vi "Day 3 - Rucksack Reorganization.vi"() -> ()   [LabVIEW 2020, in "AoC 2022.lvlib"]
uses:
  AoC 2022.lvlib
  ce42cd03-0f94-4c27-a141-a346cd3f8d99.vi
  cd464179-cc1e-4cd7-81b7-9d6a09eaff52.vi
panel:
  out "Puzzle Part-2 Answer":string
  out "Puzzle Answer":string
  in  "Puzzle Input":string
  # "Enter the Puzzle Input and run the VI"
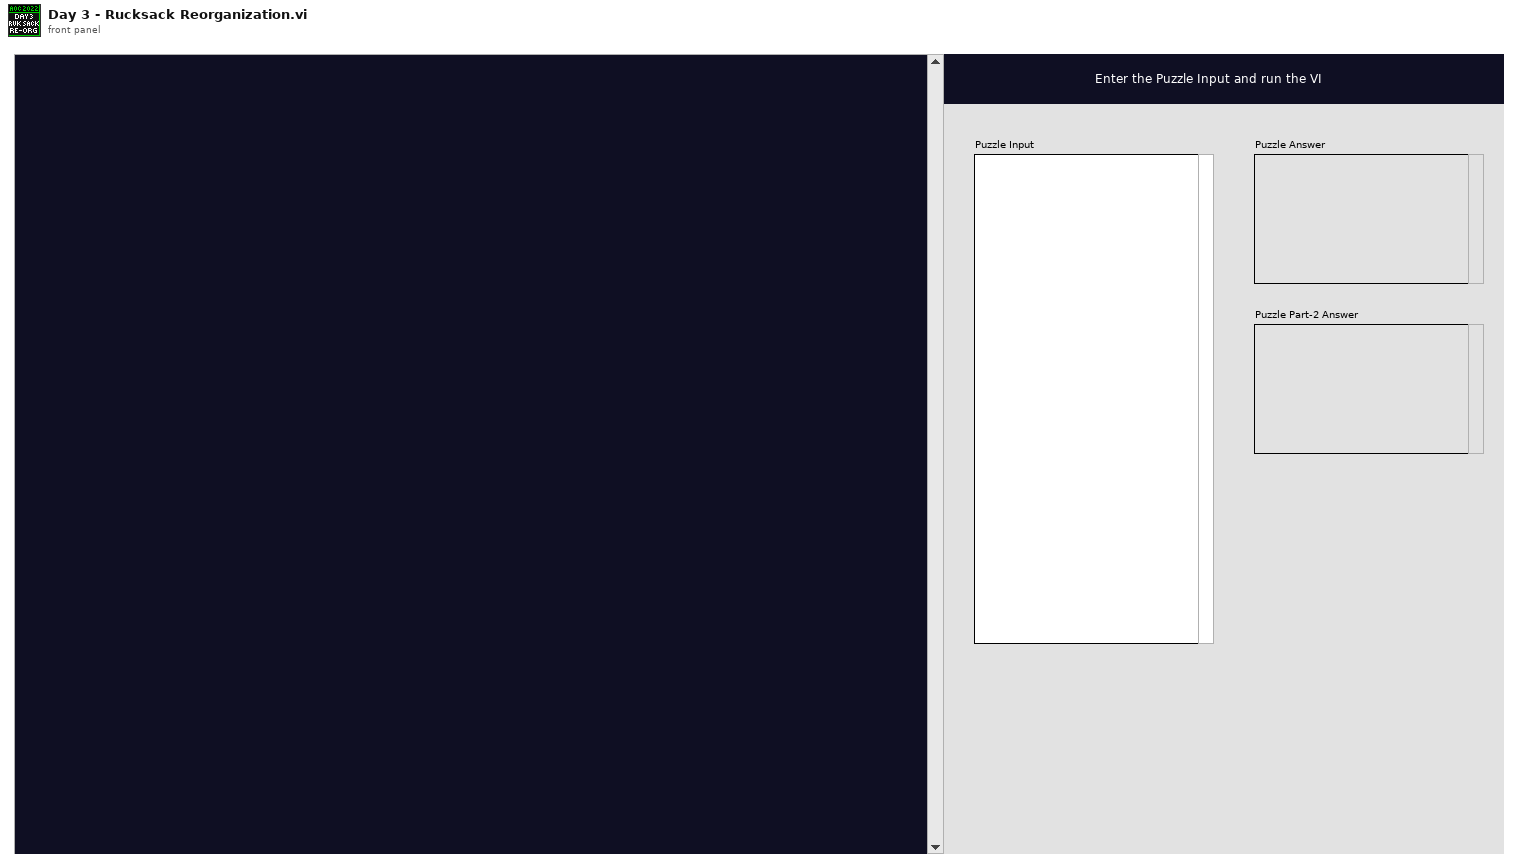
[diagram p1: front panel]
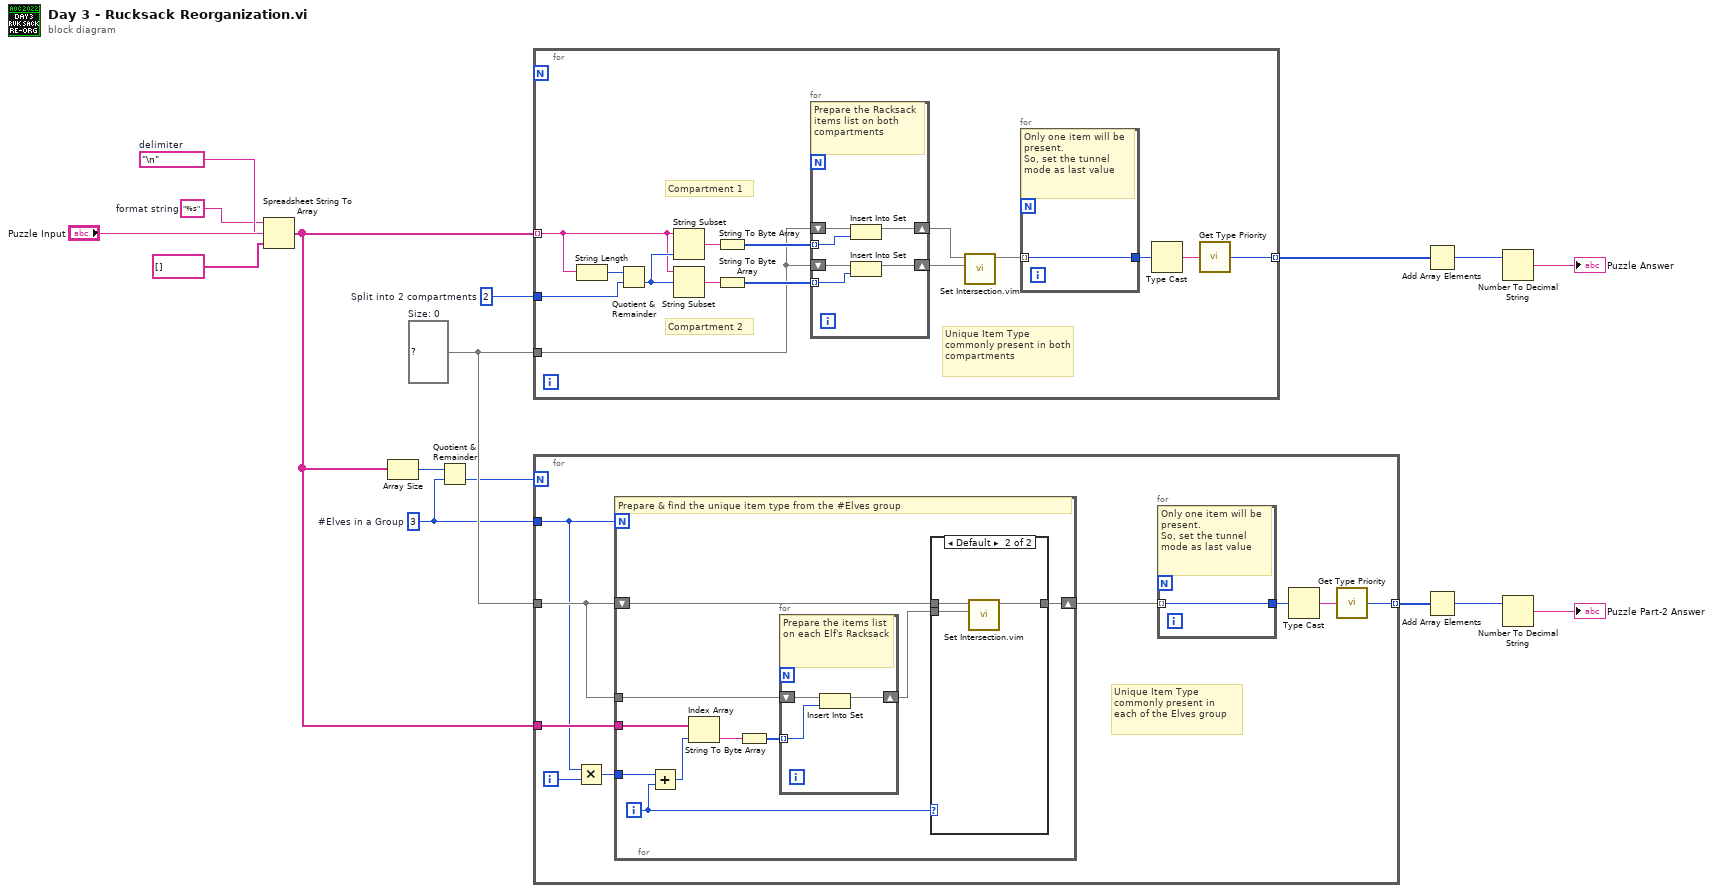
[diagram p0: block diagram]
diagram:
  w2 = 3  # #Elves in a Group
  w6 = set{u8} {}  # Size: 0
  w7 = 2  # Split into 2 compartments
  w14 = "%s"  # format string
  w15 = "\n"  # delimiter
  n1 = Spreadsheet String To Array(delimiter (Tab)=w15, format string=w14, spreadsheet string="Puzzle Input", array type (2D Dbl)=string[] []) -> (array=w5:string[])
  n2 = Array Size(array=w5) -> (size(s)=w4:i32)
  n3 = Quotient & Remainder(x=w4, y=w2) -> (floor(x/y)=w3:i32)  [unwired: 1 out]
  n4 = for {
    tunnel: w5 -> [w17] mode=indexing
    tunnel: [w18] -> w12 mode=indexing
    tunnel: w7 -> [w30]
    tunnel: w6 -> [w24]
    # "Compartment 2"
    # "Compartment 1"
    # "Unique Item Type commonly present in both compartments"
    n5 = String Length(string=w17) -> (length=w31:i32)
    n6 = Quotient & Remainder(x=w31, y=w30) -> (floor(x/y)=w29:i32)  [unwired: 1 out]
    n7 = String Subset(string=w17, length (rest)=w29) -> (substring=w28:string)  [unwired: 1 in]
    n8 = String Subset(string=w17, offset (0)=w29) -> (substring=w27:string)  [unwired: 1 in]
    n9 = String To Byte Array(string=w28) -> (unsigned byte array=w26:u8[])
    n10 = String To Byte Array(string=w27) -> (unsigned byte array=w25:u8[])
    n11 = for {
      tunnel: w26 -> [w38] mode=indexing
      tunnel: w25 -> [w35] mode=indexing
      shift-right: [w37] -> w23
      shift-left: w24 -> [w36]
      shift-right: [w34] -> w22
      shift-left: w24 -> [w33]
      # "Prepare the Racksack items list on both compartments"
      n12 = Insert Into Set(10:w38, 11:w36) -> (3:w37:set{u8})  [unwired: 1 out]
      n13 = Insert Into Set(10:w35, 11:w33) -> (3:w34:set{u8})  [unwired: 1 out]
    }
    n14 = call "Set Intersection.vim"("set 2"=w22, "set 1"=w23) -> ("intersection"=w21:set{u8})  [unwired: 9 in]
    n15 = for {
      tunnel: w21 -> [w32] mode=indexing
      tunnel: [w32] -> w19
      # "Only one item will be present.\nSo, set the tunnel mode as last value"
    }
    n16 = Type Cast(x=w19) -> (*(type *) &x=w20:string)  [unwired: 1 in]
    n17 = call "Get Type Priority.vi"("Item Type"=w20) -> ("Priority"=w18:u32)  [unwired: 4 in]
  }
  n18 = for {
    N: w3 -> [_]
    tunnel: w5 -> [w42]
    tunnel: [w44] -> w1 mode=indexing
    tunnel: w6 -> [w43]
    tunnel: w2 -> [w40]
    i -> [w41]
    # "Unique Item Type commonly present in each of the Elves group"
    n19 = Multiply(x=w40, y=w41) -> (x*y=w39:i32)
    n20 = for {
      N: w40 -> [_]
      shift-right: [w56] -> w47
      shift-left: w43 -> [w53]
      tunnel: w43 -> [w54]
      tunnel: w42 -> [w52]
      tunnel: w39 -> [w50]
      i -> [w48]
      # "Prepare & find the unique item type from the #Elves group"
      n21 = Add(x=w50, y=w48) -> (x+y=w49:i32)
      n22 = Index Array(array=w52, index=w49) -> (element=w51:string)
      n23 = String To Byte Array(string=w51) -> (unsigned byte array=w57:u8[])
      n24 = for {
        tunnel: w57 -> [w64] mode=indexing
        shift-right: [w63] -> w55
        shift-left: w54 -> [w62]
        # "Prepare the items list on each Elf's Racksack"
        n25 = Insert Into Set(10:w64, 11:w62) -> (3:w63:set{u8})  [unwired: 1 out]
      }
      n26 = case shown="Default" w48 {
        tunnel: [w58 w61] -> w56
        tunnel: w55 -> [w58 w60]
        tunnel: w53 -> [_ w59]
        frame 0 {
          # "This is the first Elf in the group.\n\nFind the unique item types between 2 Elves.\n\nContinue finding until we reach the last Elf."
        }
        frame Default {
          n27 = call "Set Intersection.vim"("set 2"=w60, "set 1"=w59) -> ("intersection"=w61:set{u8})  [unwired: 9 in]
        }
      }
    }
    n28 = for {
      tunnel: w47 -> [w65] mode=indexing
      tunnel: [w65] -> w45
      # "Only one item will be present.\nSo, set the tunnel mode as last value"
    }
    n29 = Type Cast(x=w45) -> (*(type *) &x=w46:string)  [unwired: 1 in]
    n30 = call "Get Type Priority.vi"("Item Type"=w46) -> ("Priority"=w44:u32)  [unwired: 4 in]
  }
  n31 = Add Array Elements(numeric array=w12) -> (sum=w11:u32)
  n32 = Add Array Elements(numeric array=w1) -> (sum=w9:u32)
  n33 = Number To Decimal String(number=w11) -> (decimal integer string=→"Puzzle Answer":string)  [unwired: 1 in]
  n34 = Number To Decimal String(number=w9) -> (decimal integer string=→"Puzzle Part-2 Answer":string)  [unwired: 1 in]
